vi "Agilent 2000 3000 X-Series Waveform Generator.vi"() -> ()   [LabVIEW 2015]
doc: "This example shows how to configure and output a user specific waveform. \n\n<B>Note:</B> This example is only applicable for the models which have the waveform generator license."
uses:
  <instrlib>/Agilent 2000 3000 X-Series/Agilent 2000 3000 X-Series.lvlib
panel:
  in  "Enable Output (F: Disable)":bool
  in  "Offset (0.0 V)":dbl
  in  "Amplitude (1.0 V)":dbl=1.0
  in  "Frequency (1000 Hz)":dbl=1000.0
  in  "Function Type (0: Sine)":i32(ring) items=["Sine", "Square", "Ramp", "Pulse", "Noise", "DC"]
  in  "VISA resource name":refnum<visa-resource-name>
  # "(c) 2011-2016 National Instruments.  ALL RIGHTS RESERVED."
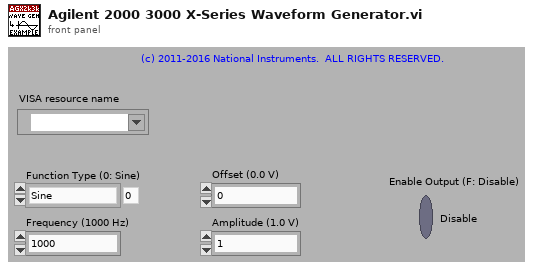
[diagram p1: front panel]
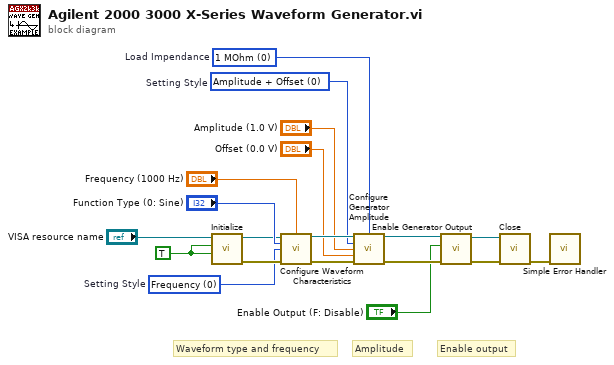
[diagram p0: block diagram]
diagram:
  w9 = 0 items=["1 MOhm", "50 Ohm"]  # Load Impendance
  w10 = 0 items=["Amplitude + Offset", "High Level + Low Level"]  # Setting Style
  w12 = 0 items=["Frequency", "Period"]  # Setting Style
  w18 = TRUE ("ID Query (True)")
  # "Enable output"
  # "Amplitude"
  # "Waveform type and frequency"
  n1 = call <instrlib>:"Initialize.vi"("Reset (True)"=w18, "ID Query (True)"=w18, "VISA resource name"="VISA resource name") -> ("error out"=w14:errorcluster, "VISA resource name out"=w15:refnum<visa-resource-name>)  [unwired: 1 in, 6 out]
  n2 = call <instrlib>:"Configure Waveform Characteristics.vi"("VISA resource name"=w15, "Frequency (1000 Hz)"="Frequency (1000 Hz)", "Function Type (0: Sine)"="Function Type (0: Sine)", "Setting Style (0: Frequency)"=w12, "error in (no error)"=w14) -> ("VISA resource name out"=w16:refnum<visa-resource-name>, "error out"=w11:errorcluster)  [unwired: 6 in, 3 out]
  n3 = call <instrlib>:"Configure Generator Amplitude.vi"("VISA resource name"=w16, "Load Impendance (0: 1 MOhm)"=w9, "Setting Style (0: Amplitude + Offset)"=w10, "Amplitude (1.0 V)"="Amplitude (1.0 V)", "Offset (0.0 V)"="Offset (0.0 V)", "error in (no error)"=w11) -> ("VISA resource name out"=w6:refnum<visa-resource-name>, "error out"=w5:errorcluster)  [unwired: 3 in, 5 out]
  n4 = call <instrlib>:"Enable Generator Output.vi"("error in (no error)"=w5, "Enable Output (F: Disable)"="Enable Output (F: Disable)", "VISA resource name"=w6) -> ("error out"=w2:errorcluster, "VISA resource name out"=w3:refnum<visa-resource-name>)  [unwired: 1 in, 6 out]
  n5 = call <instrlib>:"Close.vi"("error in (no error)"=w2, "VISA resource name"=w3) -> ("error out"=w1:errorcluster)  [unwired: 9 out]
  n6 = call <vilib>:"Simple Error Handler.vi"("error in (no error)"=w1) -> ()  [unwired: 1 in, 8 out]
